vi "TCP_comms_test_send.vi"() -> ()   [LabVIEW 2018]
panel:
  out "Sent i":i32
  in  "Send many":bool
  in  "Value to send":u32
  in  "Send single value":bool
  out "Error Out":errorcluster
  in  "Stop and Exit":bool
  in  "Error In":errorcluster
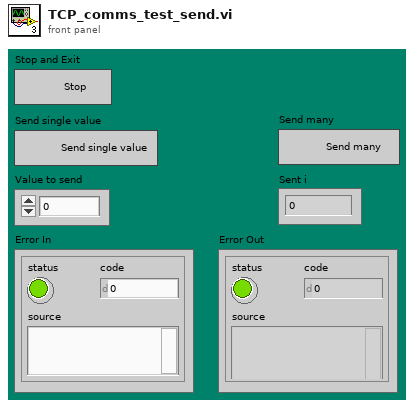
[diagram p1: front panel]
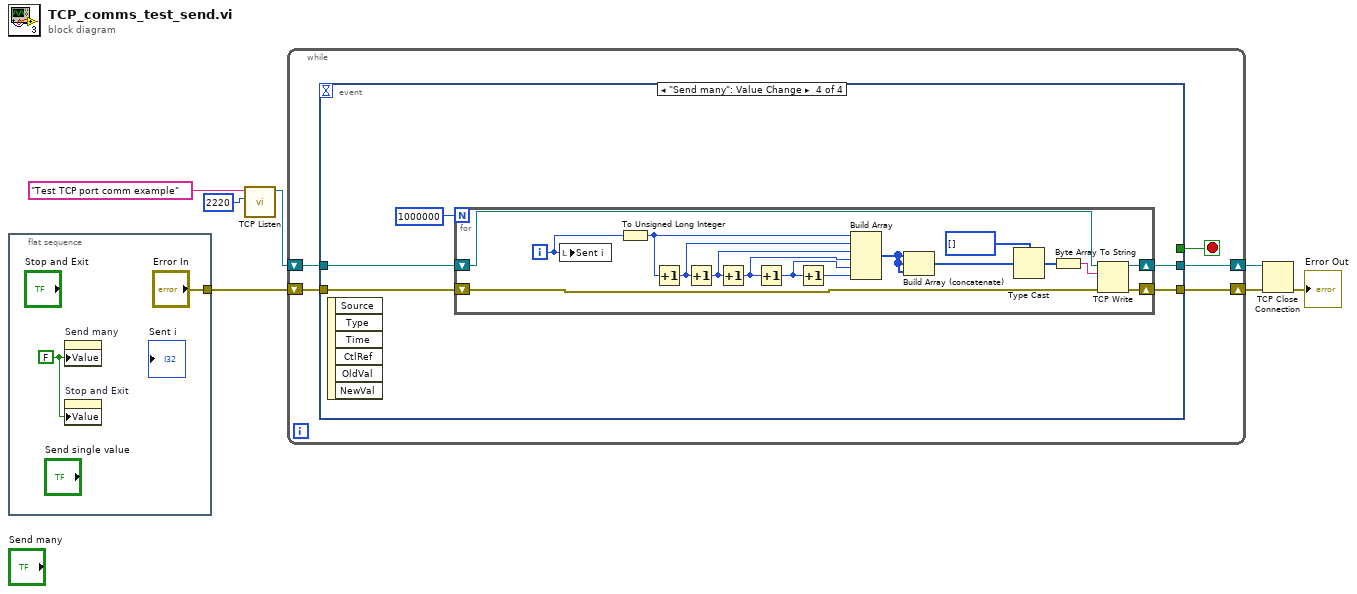
[diagram p0: block diagram]
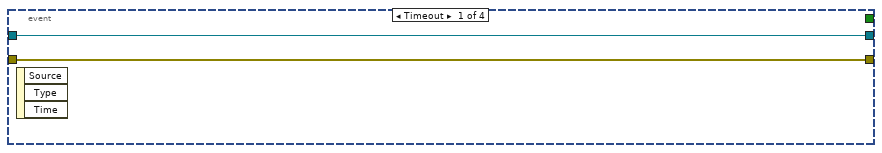
[diagram p2: hidden frame]
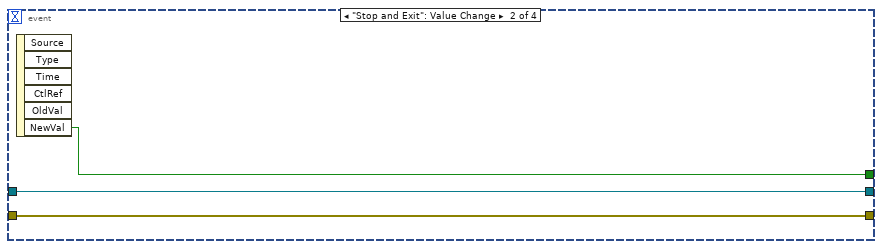
[diagram p3: hidden frame]
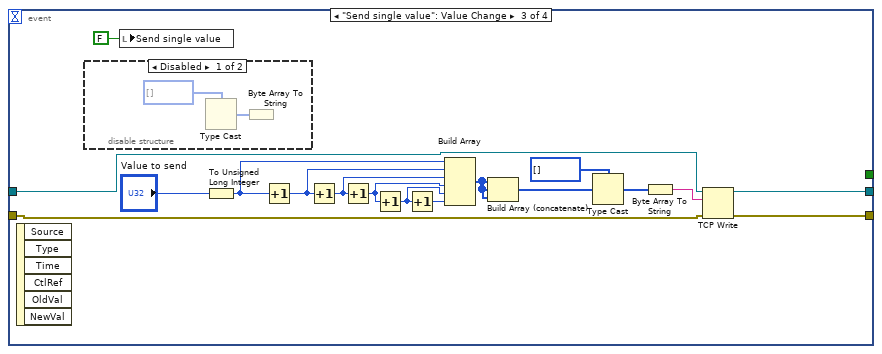
[diagram p4: hidden frame]
diagram:
  n1 = flat-sequence {
    tunnel: ["Error In"] -> w7
    frame #0 {
      w8 = FALSE ("Stop and Exit")
      n2 = property on="Send many" class="Bool (strict)"("Value"=w8) -> ()  [unwired: 2 in, 2 out]
      n3 = property on="Stop and Exit" class="Bool (strict)"("Value"=w8) -> ()  [unwired: 2 in, 2 out]
    }
  }
  n4 = call <vilib>:"TCP Listen.vi"("port"=u16 2220, "service name"="Test TCP port comm example") -> ("connection ID"=w2:refnum<k5>)  [unwired: 5 in, 4 out]
  n5 = while {
    shift-right: [w12] -> w6
    shift-left: w7 -> [w13]
    shift-right: [w10] -> w5
    shift-left: w2 -> [w11]
    stop <- w14 stop-if-true
    n6 = event shown="[3] \"Send many\": Value Change" {
      selector: _ -> [_ _ _ _]
      dyn-events: _ -> [_ _ _ _]
      timeout: _ -> [_ _ _ _]
      tunnel: [_ w19 _ _] -> w14
      tunnel: w13 -> [w16 w18 w34 w42]
      tunnel: [w16 w18 w33 w41] -> w12
      tunnel: w11 -> [w15 w17 w36 w44]
      tunnel: [w15 w17 w35 w43] -> w10
      event Timeout {
        n7 = event-data() -> ()  [unwired: 1 in, 3 out]
      }
      event "Stop and Exit": Value Change {
        n8 = event-data() -> ("NewVal"=w19:bool)  [unwired: 1 in, 5 out]
      }
      event "Send single value": Value Change {
        n9 = event-data() -> ()  [unwired: 1 in, 6 out]
        n10 = disable-structure shown="Disabled" {
          frame Disabled {
            n11 = Type Cast(type=u8[] []) -> (x=w39:ext, *(type *) &x=w38:u8[])
            n12 = Byte Array To String(unsigned byte array=w38) -> ()  [unwired: 1 out]
          }
          frame Enabled {
          }
        }
        n13 = local write "Send single value"(FALSE ("Send single value")) -> ()
        n14 = To Unsigned Long Integer(number="Value to send") -> (unsigned 32bit integer=w28:u32)
        n15 = Increment(x=w28) -> (x+1=w27:u32)
        n16 = Increment(x=w27) -> (x+1=w26:u32)
        n17 = Increment(x=w26) -> (x+1=w25:u32)
        n18 = Increment(x=w25) -> (x+1=w24:u32)
        n19 = Increment(x=w24) -> (x+1=w23:u32)
        n20 = Build Array(w28, w27, w26, w25, w24, w23) -> (w21:u32[])
        n21 = Build Array (concatenate)(w21, w21, w21) -> (w20:u32[])
        n22 = Type Cast(type=u8[] [], x=w20) -> (*(type *) &x=w31:u8[])
        n23 = Byte Array To String(unsigned byte array=w31) -> (string=w30:string)
        n24 = TCP Write(connection ID=w36, data in=w30, error in (no error)=w34) -> (connection ID out=w35:refnum<k5>, error out=w33:errorcluster)  [unwired: 1 in, 1 out]
      }
      event "Send many": Value Change {
        n25 = event-data() -> ()  [unwired: 1 in, 6 out]
        n26 = for {
          N: 1000000 -> [_]
          shift-right: [w59] -> w43
          shift-left: w44 -> [w60]
          shift-right: [w57] -> w41
          shift-left: w42 -> [w58]
          i -> [w45]
          n27 = local write "Sent i"(w45) -> ()
          n28 = To Unsigned Long Integer(number=w45) -> (unsigned 32bit integer=w53:u32)
          n29 = Increment(x=w53) -> (x+1=w52:u32)
          n30 = Increment(x=w52) -> (x+1=w51:u32)
          n31 = Increment(x=w51) -> (x+1=w50:u32)
          n32 = Increment(x=w50) -> (x+1=w49:u32)
          n33 = Increment(x=w49) -> (x+1=w48:u32)
          n34 = Build Array(w53, w52, w51, w50, w49, w48) -> (w47:u32[])
          n35 = Build Array (concatenate)(w47, w47, w47) -> (w46:u32[])
          n36 = Type Cast(type=u8[] [], x=w46) -> (*(type *) &x=w55:u8[])
          n37 = Byte Array To String(unsigned byte array=w55) -> (string=w54:string)
          n38 = TCP Write(connection ID=w60, data in=w54, error in (no error)=w58) -> (connection ID out=w59:refnum<k5>, error out=w57:errorcluster)  [unwired: 1 in, 1 out]
        }
      }
    }
  }
  n39 = TCP Close Connection(connection ID=w5, error in (no error)=w6) -> (error out=→"Error Out":errorcluster)  [unwired: 1 in, 1 out]
